vi "DAC Save Results.vi"(8 "error in":errorcluster, 9 "Log Details?":bool, 10 "tdms file":refnum<k34>, 11 "DAC in":refnum<class "DAC.lvclass">) -> (0 "error out":errorcluster)   [LabVIEW 2019, in "DAC.lvlib" / "DAC.lvclass"]
uses:
  DAC.lvclass
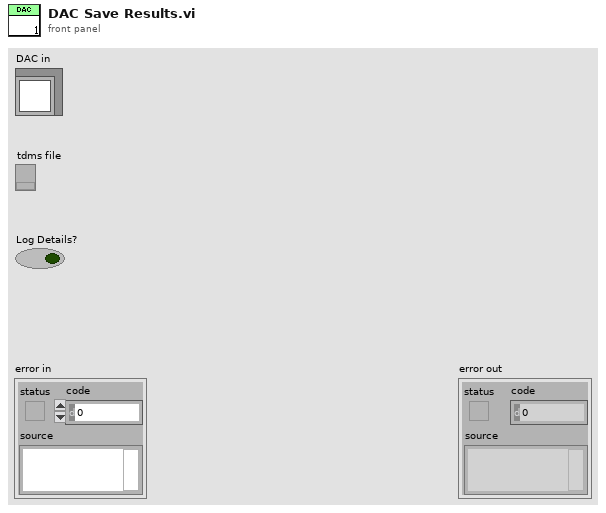
[diagram p1: front panel]
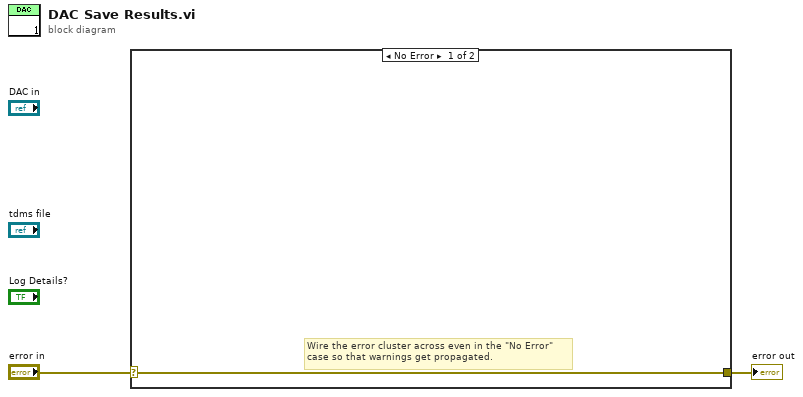
[diagram p0: block diagram]
diagram:
  n1 = case shown="No Error" "error in" {
    selector: "error in" -> [w3 w4]
    tunnel: [w3 w4] -> w1
    frame No Error {
      # "Wire the error cluster across even in the \"No Error\"\ncase so that warnings get propagated."
    }
    frame Error {
    }
  }
  "error out" <- w1
